vi "Get VISA gRPC Open Close Behavior.vi"(8 "error in (no error)":errorcluster, 11 "initialize session behavior":T2) -> (0 "error out":errorcluster, 3 "open/close behavior":T1)   [LabVIEW 2020, in "Keysight 34401A DMM Instrument.lvlib" / "Session Factory.lvclass"]
uses:
  Session Factory.lvclass
  <vilib>/NI-VISA/VISA gRPC Open Close Behavior.ctl
  <vilib>/Plug-In SDKs/Sessions/Instrument/ISession Factory/Initialize and Close Session Behavior.ctl
  <vilib>/Plug-In SDKs/Sessions/Instrument/ISession Factory/ISession Factory.lvclass
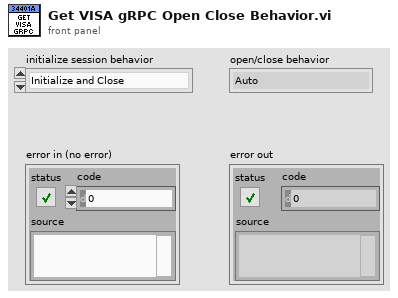
[diagram p1: front panel]
types:
  T1 = typedef "VISA gRPC Open Close Behavior.ctl" = enum16{"Auto", "Initialize and Close", "Attach and Detach", "Initialize and Detach", "Attach and Close"}
  T2 = typedef "NI Session Management Instrument.lvlib/ISession Factory.lvclass/Initialize and Close Session Behavior.ctl" = enum16{"Initialize and Close", "Attach and Detach", "Initialize and Detach", "Attach and Close"}
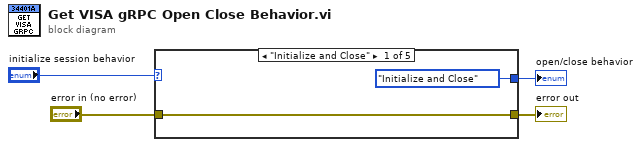
[diagram p0: block diagram]
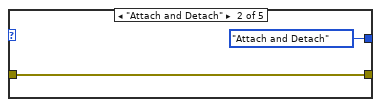
[diagram p2: hidden frame]
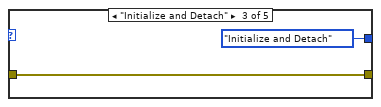
[diagram p3: hidden frame]
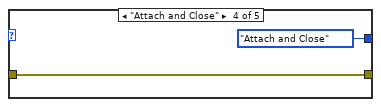
[diagram p4: hidden frame]
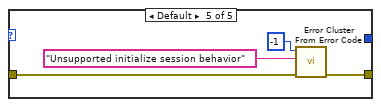
[diagram p5: hidden frame]
diagram:
  n1 = case shown="\"Initialize and Close\"" "initialize session behavior" {
    tunnel: [VISA_gRPC_Open_Close_Behavior."Initialize and Close" ("open/close behavior") VISA_gRPC_Open_Close_Behavior."Attach and Detach" ("open/close behavior") VISA_gRPC_Open_Close_Behavior."Initialize and Detach" ("open/close behavior") VISA_gRPC_Open_Close_Behavior."Attach and Close" ("open/close behavior") _] -> w3
    tunnel: [w5 w7 w9 w11 w15] -> w2
    tunnel: "error in (no error)" -> [w5 w7 w9 w11 w16]
    frame "Initialize and Close" {
    }
    frame "Attach and Detach" {
    }
    frame "Initialize and Detach" {
    }
    frame "Attach and Close" {
    }
    frame Default {
      n2 = call <vilib>:"Error Cluster From Error Code.vi"("error in (no error)"=w16, "error message (\"\")"="Unsupported initialize session behavior" ("error message (\"\")"), "error code (0)"=-1) -> ("error out"=w15:errorcluster)  [unwired: 6 in]
    }
  }
  "open/close behavior" <- w3
  "error out" <- w2
